vi "HF turbidimeter (com4).vi"(4 "State":i16, 5 "Time":dbl format="%.2f", 6 "Sensor Values":dbl[](array[numeric]), 7 "Set Points":dbl[](array[numeric])) -> (0 "required data":T2={"Set Point names"=["unitID (usually 1)"], "required number of setpoints"=1, "required number of sensors"=0, "Sensor names"=[]}, 3 "output value":dbl)   [LabVIEW 2012]
uses:
  <vilib>/Instr/_visa.llb/VISA Configure Serial Port (Instr).vi
panel:
  out "Previous data":T1(array[cluster])
  out "all bad":bool
  out "x-1":i32
  out "UnitID":i32
  out "write buffer":string
  out "Numeric":i32
  # "Enter the correct information for this control code in the required data structure below. Then make the current value default by right clicking on the border of the data structure. Select \"data operations\" and then select \"make current value default\". These values will be displayed by process controller."
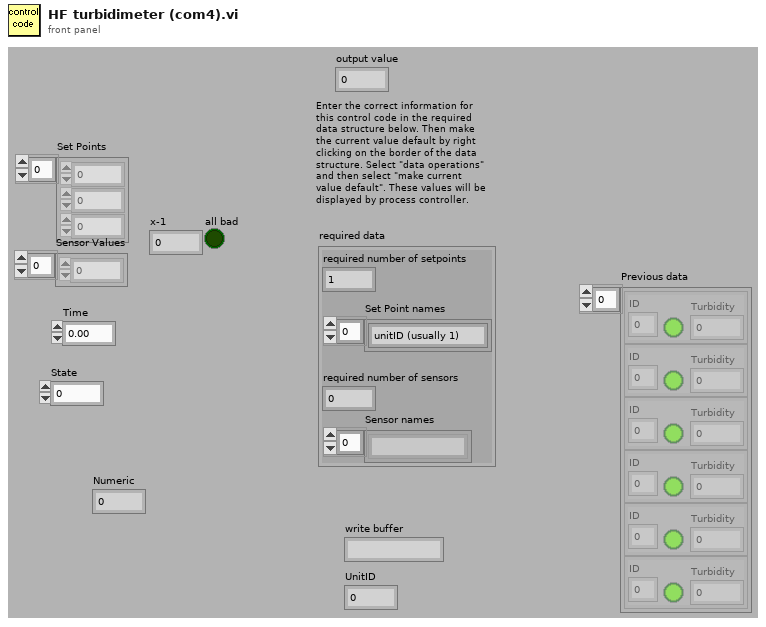
[diagram p1: front panel]
types:
  T1 = cluster{"ID":dbl, "Failed":bool, "Turbidity":dbl}[]
  T2 = cluster{"Set Point names":string[], "required number of setpoints":u8, "required number of sensors":u8, "Sensor names":string[]}
  T3 = cluster{"ID":dbl, "Failed":bool, "Turbidity":dbl}
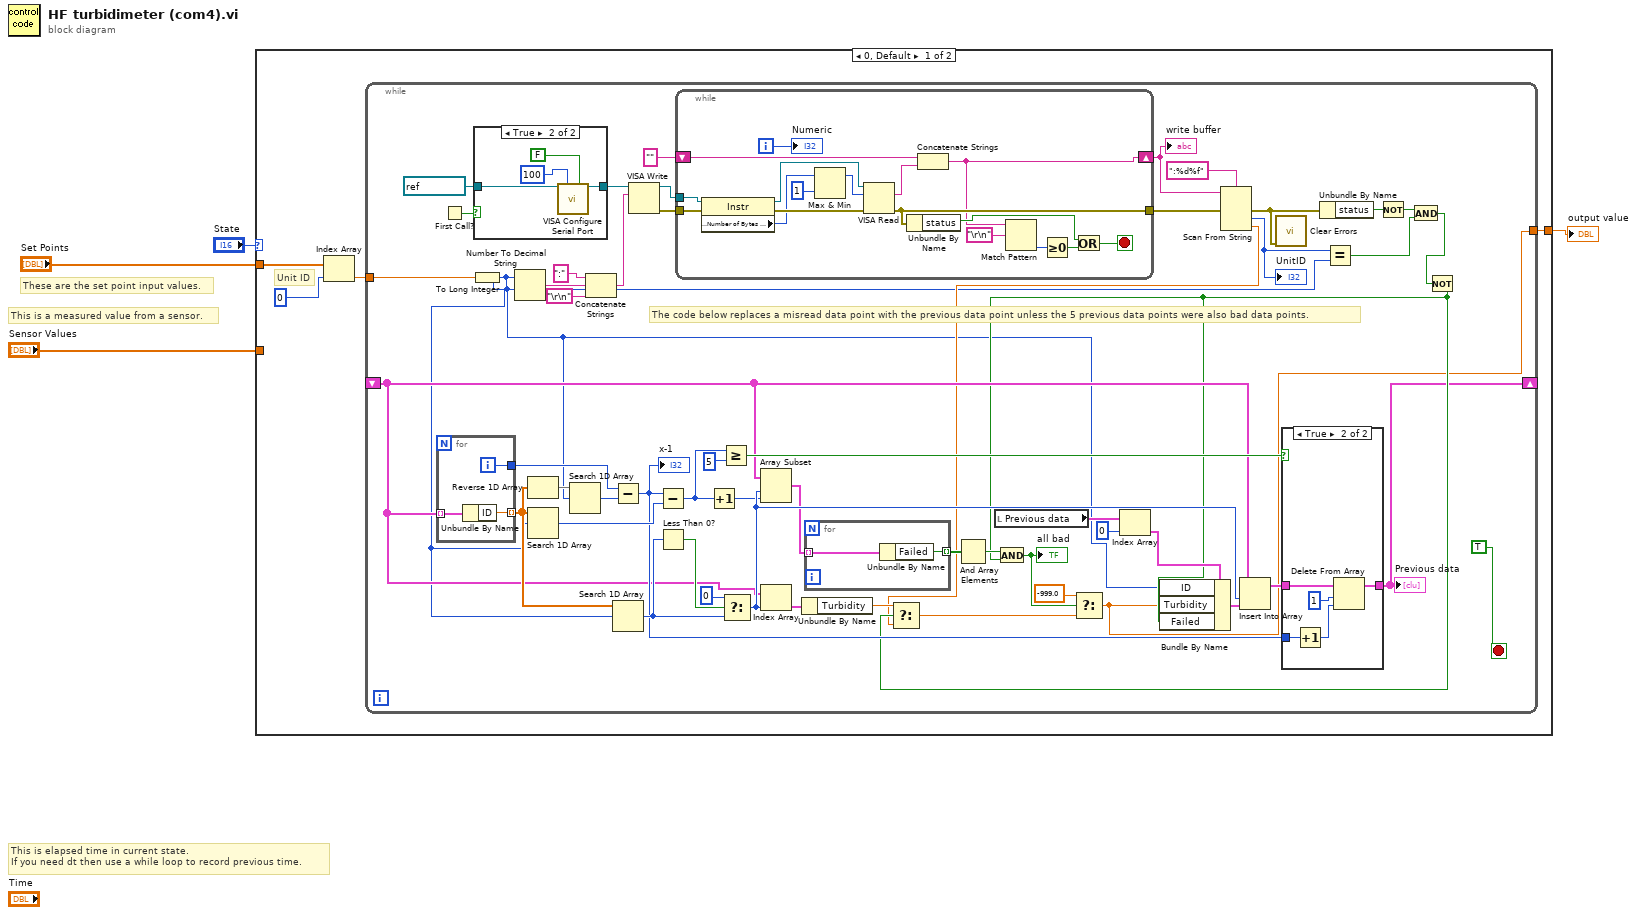
[diagram p0: block diagram]
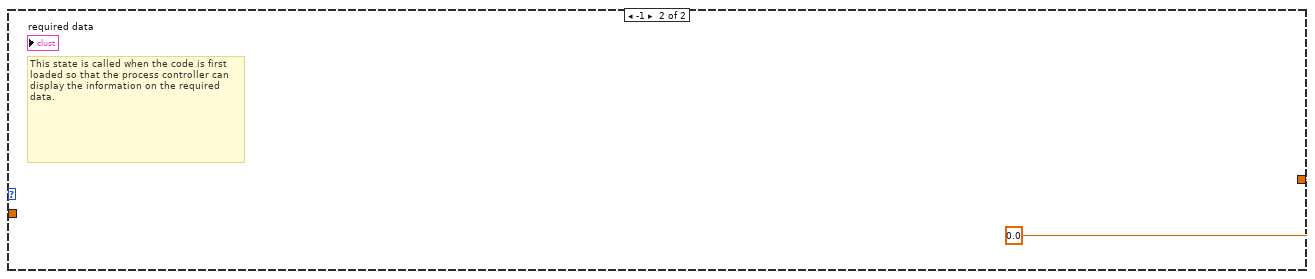
[diagram p4: hidden frame]
diagram:
  # "These are the set point input values."
  # "This is a measured value from a sensor."
  # "This is elapsed time in current state.\nIf you need dt then use a while loop to record previous time."
  n1 = case shown="0, Default" "State" {
    tunnel: [w5 0.0 ("fraction on")] -> w3
    tunnel: "Set Points" -> [w7 _]
    tunnel: "Sensor Values" -> [_ _]
    frame 0, Default {
      # "Unit ID"
      n2 = Index Array(array=w7, index=0) -> (element=w6:dbl)
      n3 = while {
        tunnel: w6 -> [w51]
        tunnel: [w10] -> w5
        shift-right: [w9] -> _
        shift-left: _ -> [w15]
        stop <- TRUE stop-if-true
        # "The code below replaces a misread data point with the previous data point unless the 5 previous data points were also bad data points."
        n4 = for {
          tunnel: w15 -> [w67] mode=indexing
          tunnel: [w66] -> w22 mode=indexing
          tunnel: [w65] -> w21
          i -> [w65]
          n5 = Unbundle By Name(w67) -> ("ID"=w66:dbl)
        }
        n6 = First Call?() -> (First Call?: T/F=w53:bool)
        n7 = To Long Integer(number=w51) -> (32bit integer=w11:i32)
        n8 = case shown="True" w53 {
          tunnel: [w74 w78] -> w61
          tunnel: refnum<visa-resource-name> "COM4" ("VISA resource name") -> [w74 w75]
          frame False {
          }
          frame True {
            n9 = call-poly "VISA Configure Serial Port"("VISA resource name"=w75, "timeout (10sec)"=u32 100, "Enable Termination\nChar (T)"=FALSE ("Enable Termination\nChar (T)")) -> ("VISA resource name out"=w78:refnum<visa-resource-name>)  [unwired: 11 in, 1 out]
          }
        }
        n10 = Number To Decimal String(number=w11) -> (decimal integer string=w54:string)  [unwired: 1 in]
        n11 = Reverse 1D Array(array=w22) -> (reversed array=w38:dbl[])
        n12 = Search 1D Array(1D array=w22, element=w11) -> (index of element=w34:i32)  [unwired: 1 in]
        n13 = Search 1D Array(1D array=w38, element=w11) -> (index of element=w37:i32)  [unwired: 1 in]
        n14 = Concatenate Strings(":" ("string"), w54, "\r\n") -> (w57:string)
        n15 = Subtract(x=w21, y=w37) -> (x-y=w28:i32)
        "x-1" <- w28
        n16 = Search 1D Array(1D array=w22, element=w11) -> (index of element=w32:i32)  [unwired: 1 in]
        n17 = VISA Write(VISA resource name=w61, write buffer=w57) -> (VISA resource name out=w60:refnum<visa-resource-name>, error out=w59:errorcluster)  [unwired: 1 in, 1 out]
        n18 = Subtract(x=w28, y=w34) -> (x-y=w25:i32)
        n19 = Less Than 0?(x=w32) -> (x < 0?=w33:bool)
        n20 = while {
          tunnel: w60 -> [w94]
          tunnel: w59 -> [w92]
          shift-right: [w79] -> w47
          shift-left: "" ("write buffer") -> [w95]
          tunnel: [w81] -> w50
          i -> [w80]
          stop <- w90 stop-if-true
          n21 = property class="Instr"(reference=w94, error in=w92) -> (reference out=w93:refnum<visa-resource-name>, error out=w91:errorcluster, "Serial Settings:Number of Bytes at Serial Port"=w83:u32)
          n22 = Max & Min(x=w83, y=u32 1) -> (max(x,y)=w84:u32)  [unwired: 1 out]
          n23 = VISA Read(VISA resource name=w93, byte count=w84, error in (no error)=w91) -> (read buffer=w88:string, error out=w81:errorcluster)  [unwired: 2 out]
          n24 = Unbundle By Name(w81) -> ("status"=w89:bool)
          n25 = Concatenate Strings(w95, w88) -> (w79:string)
          n26 = Match Pattern(string=w79, regular expression="\r\n") -> (offset past match=w86:i32)  [unwired: 1 in, 3 out]
          n27 = Greater Or Equal To 0?(x=w86) -> (x >= 0?=w85:bool)
          n28 = Or(x=w89, y=w85) -> (x .or. y?=w90:bool)
          "Numeric" <- w80
        }
        "write buffer" <- w47
        n29 = Increment(x=w25) -> (x+1=w24:i32)
        n30 = Greater Or Equal?(x=w25, y=5) -> (x >= y?=w35:bool)
        n31 = Select(t=0 ("index of element"), s=w33, f=w32) -> (s? t:f=w26:i32)
        n32 = Array Subset(array=w15, index=w26, length=w24) -> (w23:T1)
        n33 = Index Array(array=w15, index=w26) -> (element=w30:T3)
        n34 = Unbundle By Name(w30) -> ("Turbidity"=w29:dbl)
        n35 = for {
          tunnel: w23 -> [w64] mode=indexing
          tunnel: [w63] -> w20 mode=indexing
          n36 = Unbundle By Name(w64) -> ("Failed"=w63:bool)
        }
        n37 = And Array Elements(Boolean array=w20) -> (logical AND=w17:bool)
        n38 = local read "Previous data"() -> (w42:T1)
        n39 = Index Array(array=w42, index=0) -> (element=w40:T3)
        n40 = Scan From String(format string=":%d%f", input string=w47, error in=w50) -> (error out=w49:errorcluster, output 1=w46:i32, output 2=w12:dbl)  [unwired: 3 in, 2 out]
        "UnitID" <- w46
        n41 = call <vilib>:"Clear Errors.vi"("error in (no error)"=w49) -> ()  [unwired: 6 in, 1 out]
        n42 = Unbundle By Name(w49) -> ("status"=w48:bool)
        n43 = Equal?(x=w46, y=w11) -> (x = y?=w44:bool)
        n44 = Not(x=w48) -> (.not. x?=w45:bool)
        n45 = And(x=w45, y=w44) -> (x .and. y?=w14:bool)
        n46 = Not(x=w14) -> (.not. x?=w13:bool)
        n47 = Select(t=w29, s=w13, f=w12) -> (s? t:f=w18:dbl)
        n48 = And(x=w17, y=w13) -> (x .and. y?=w16:bool)
        "all bad" <- w16
        n49 = Select(t=-999.0, s=w16, f=w18) -> (s? t:f=w10:dbl)
        n50 = Bundle By Name(cluster=w40, "ID"=w11, "Turbidity"=w10, "Failed"=w13) -> (w39:T3)
        n51 = Insert Into Array(array=w15, index=w26, new element=w39) -> (w27:T1)
        n52 = case shown="True" w35 {
          tunnel: w27 -> [w68 w73]
          tunnel: [w68 w72] -> w9
          tunnel: w28 -> [_ w71]
          frame False {
          }
          frame True {
            n53 = Increment(x=w71) -> (x+1=w69:i32)
            n54 = Delete From Array(array=w73, length=1, index=w69) -> (array with subset deleted=w72:T1)  [unwired: 1 out]
          }
        }
        "Previous data" <- w9
      }
    }
    frame -1 {
      # "This state is called when the code is first loaded so that the process controller can display the information on the required data."
    }
  }
  "output value" <- w3
